vi "S2C_STEP_ParseCmd.vi"(8 "Error In":errorcluster, 10 "Row":i32, 11 "Data In":string[][](array[string])) -> (0 "Error Out":errorcluster, 1 "New?":bool, 2 "Settings":string[][](array[string]), 3 "Step Name":string)   [LabVIEW 2015]
doc: "Parses a Fornax JSON string and returns the text values for each parameter."
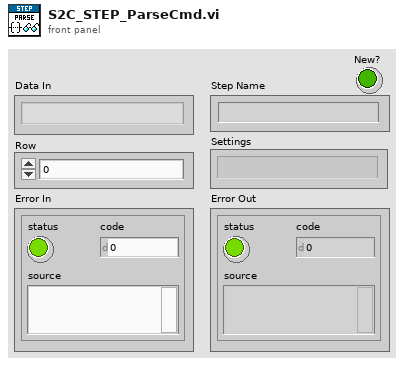
[diagram p1: front panel]
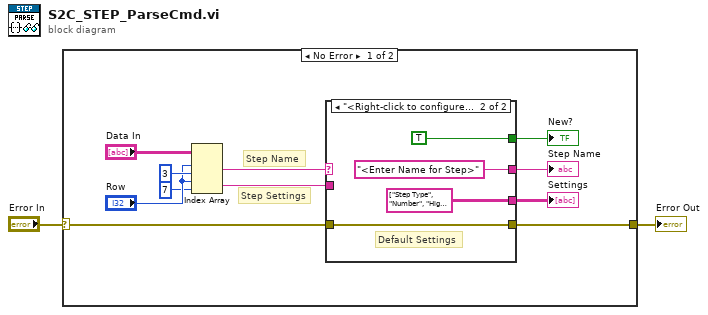
[diagram p0: block diagram]
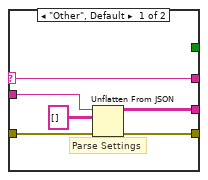
[diagram p2: hidden frame]
diagram:
  n1 = case shown="No Error" "Error In" {
    selector: "Error In" -> [w12 w24]
    tunnel: [w6 w24] -> w1
    frame No Error {
      # "Step Settings"
      # "Step Name"
      n2 = Index Array(array="Data In", index (row) #1="Row", index (col) #1=3 ("disabled index (col)"), index (row) #2="Row", index (col) #2=7 ("disabled index (col)")) -> (element #1=w5:string, element #2=w7:string)
      n3 = case shown="\"<Right-click to configure>\"" w5 {
        selector: w5 -> [w14 _]
        tunnel: [w18 string[][] [["Step Type", "Number"], ["High Limit", "10"], ["High Limit Comparison", "LE"], ["Low Limit", "0"], ["Low Limit Comparison", "GE"], ["Units", "None"], ["Log Step", "False"], ["Record Step", "True"]] ("Number")] -> w13
        tunnel: w12 -> [w17 w23]
        tunnel: w7 -> [w16 _]
        tunnel: [w15 w23] -> w6
        tunnel: [w14 "<Enter Name for Step>"] -> w4
        tunnel: [_ TRUE] -> w3
        frame "Other", Default {
          # "Parse Settings"
          n4 = Unflatten From JSON(JSON string=w16, type and defaults=string[][] [], error in (no error)=w17) -> (value=w18:string[][], error out=w15:errorcluster)  [unwired: 4 in]
        }
        frame "<Right-click to configure>" {
          # "Default Settings"
        }
      }
      "Settings" <- w13
      "Step Name" <- w4
      "New?" <- w3
    }
    frame Error {
    }
  }
  "Error Out" <- w1
